vi "time_between.vi"(0 "Y":dbl[](array[numeric]), 5 "Amplitude(V)":dbl, 7 "First value":dbl, 9 "Second Value":dbl, 11 "index":i32) -> (4 "Numeric":dbl)   [LabVIEW 2023]
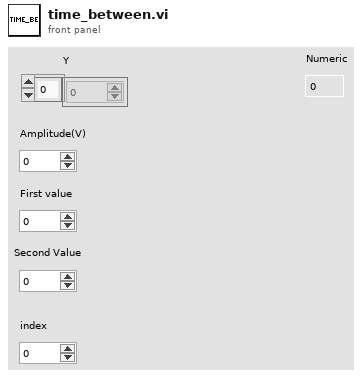
[diagram p1: front panel]
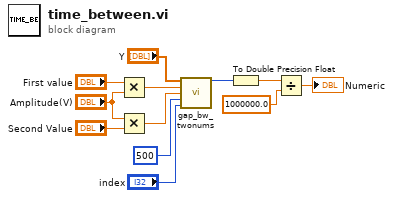
[diagram p0: block diagram]
diagram:
  n1 = Multiply(x="First value", y="Amplitude(V)") -> (x*y=w1:dbl)
  n2 = Multiply(x="Amplitude(V)", y="Second Value") -> (x*y=w2:dbl)
  n3 = call "gap_bw_twonums.vi"("Y"="Y", "element 1"=w1, "element 2"=w2, "length"=500, "index"="index") -> ("Numeric"=w3:i32)  [unwired: 8 in, 2 out]
  n4 = To Double Precision Float(number=w3) -> (double precision float=w4:dbl)
  n5 = Divide(x=w4, y=1000000.0) -> (x/y=→"Numeric":dbl)
